vi "Write Measured Table Reference.vi"(8 "error in (no error)":errorcluster, 10 "Measured Table Reference":refnum<vi>, 11 "AnalogInput in":refnum<class "AnalogInput.lvclass">) -> (0 "error out":errorcluster, 3 "AnalogInput out":refnum<class "AnalogInput.lvclass">)   [LabVIEW 2019, in "AnalogInput.lvlib" / "AnalogInput.lvclass"]
uses:
  Library/AnalogInput.lvclass
  Library/AnalogInput.lvclass/AnalogInput.ctl
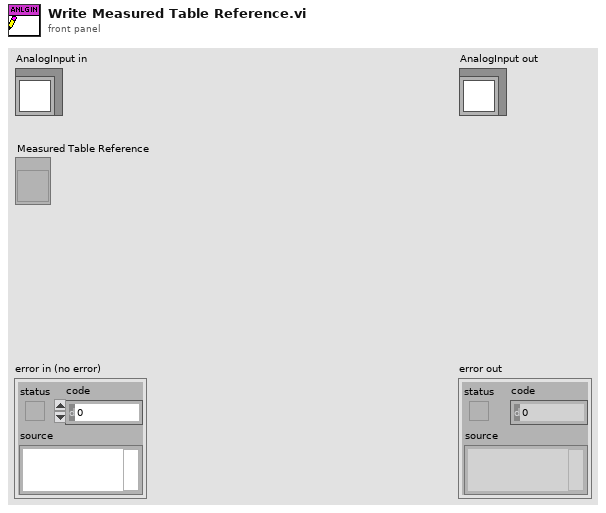
[diagram p1: front panel]
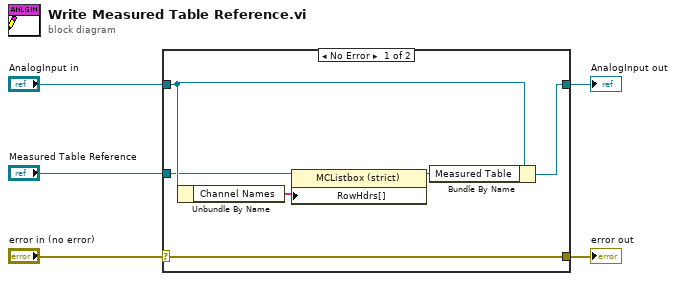
[diagram p0: block diagram]
diagram:
  n1 = case shown="No Error" "error in (no error)" {
    selector: "error in (no error)" -> [w11 w12]
    tunnel: [w11 w12] -> w4
    tunnel: [w10 w13] -> w2
    tunnel: "AnalogInput in" -> [w9 w13]
    tunnel: "Measured Table Reference" -> [w8 _]
    frame No Error {
      n2 = Unbundle By Name(w9) -> ("Channel Names"=w6:string[])
      n3 = property class="MCListbox (strict)"(reference=w8, "RowHdrs[]"=w6) -> (reference out=w7:refnum<vi>)  [unwired: 1 in, 1 out]
      n4 = Bundle By Name(cluster=w9, "Measured Table"=w7) -> (w10:refnum<class "AnalogInput.lvclass">)
    }
    frame Error {
    }
  }
  "error out" <- w4
  "AnalogInput out" <- w2
